vi "Read Tab Layout.vi"(9 "Tab in":refnum<class "Tab.lvclass">) -> (3 "Tab out":refnum<class "Tab.lvclass">, 4 "Tab Layout":T1(ring))   [LabVIEW 2014, in "Tab.lvclass"]
uses:
  Tab.lvclass
  Tab.lvclass/Tab.ctl
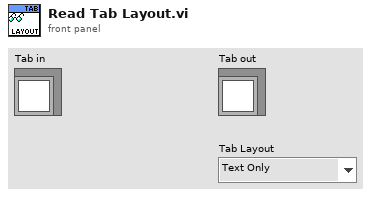
[diagram p1: front panel]
types:
  T1 = enum32{"Text Only", "Image Only", "Text - Image", "Image - Text"}
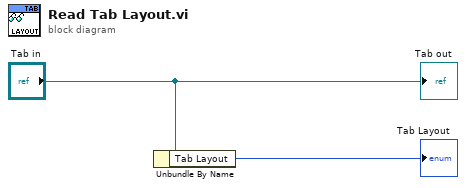
[diagram p0: block diagram]
diagram:
  n1 = Unbundle By Name("Tab in") -> ("Tab Layout"=→"Tab Layout":T1)
  "Tab out" <- "Tab in"
